vi "Start SSH Module.vi"(7 "Run as Singleton? (F)":bool, 8 "error in (no error)":errorcluster, 10 "Connection Info":T1={"host IP"="", "port"=22, "username"="lanforge", "password"="lanforge", "Connection Name"=""}) -> (0 "error out":errorcluster, 2 "Module ID":i32, 5 "SSH Broadcast Events":T2)   [LabVIEW 2017]
doc: "Creates a new instance of an SSH client with the login details specified.\nIf \"Run as Singleton\" is set to true, only one instance of the client may be created.\nRecord \"SSH Broadcast Events\" if you want to register for updates from the SSH client.\nRecord Module ID (or Connection Name) to talk to the module in future."
uses:
  Libraries/SSH/Did Init Argument--cluster.ctl
  Libraries/SSH/Status Updated Argument--cluster.ctl
  Libraries/SSH/Error Reported Argument--cluster.ctl
  Libraries/SSH/Stop Argument--cluster.ctl
  Libraries/SSH/Get Module Execution Status Argument--cluster.ctl
  Libraries/SSH/Connection Info.ctl
  Libraries/SSH/SSH.lvlib
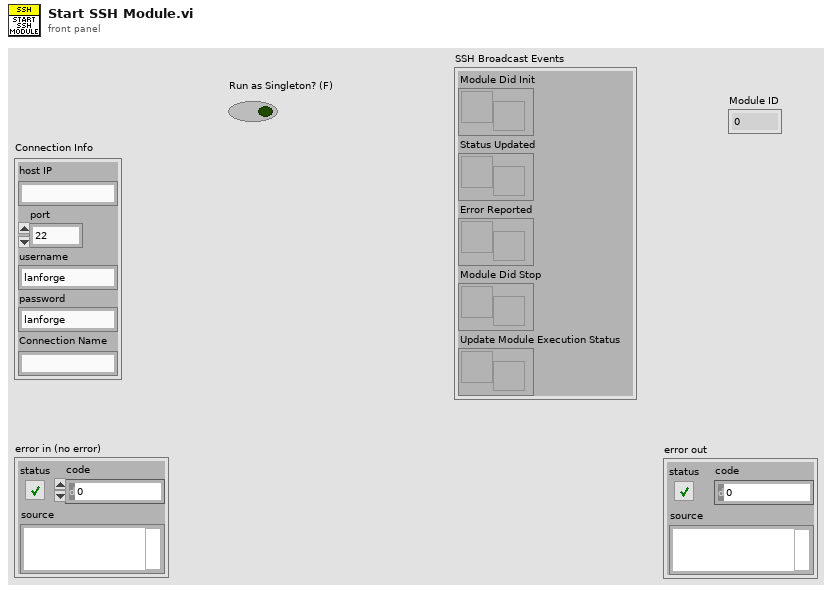
[diagram p1: front panel]
types:
  T1 = typedef "SSH.lvlib/Connection Info.ctl" = cluster{"host IP":string, "port":i32, "username":string, "password":string, "Connection Name":string}
  T2 = cluster{"Module Did Init":refnum<user-event>, "Status Updated":refnum<user-event>, "Error Reported":refnum<user-event>, "Module Did Stop":refnum<user-event>, "Update Module Execution Status":refnum<user-event>}
  T3 = typedef "SSH.lvlib/Broadcast Events--cluster.ctl" = cluster{"Module Did Init":refnum<user-event>, "Status Updated":refnum<user-event>, "Error Reported":refnum<user-event>, "Module Did Stop":refnum<user-event>, "Update Module Execution Status":refnum<user-event>}
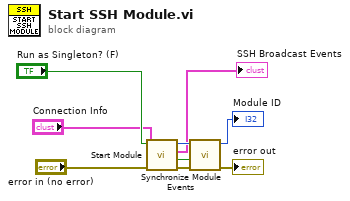
[diagram p0: block diagram]
diagram:
  n1 = call "Start Module.vi"("error in (no error)"="error in (no error)", "Connection Info"="Connection Info", "Run as Singleton? (F)"="Run as Singleton? (F)") -> ("error out"=w8:errorcluster, "Wait for Event Sync?"=w7:bool, "SSH Broadcast Events"=→"SSH Broadcast Events":T3, "Module ID"=w9:i32)  [unwired: 5 in]
  n2 = call "Synchronize Module Events.vi"("error in (no error)"=w8, "Wait for Event Sync?"=w7, "Module ID"=w9) -> ("error out"=→"error out":errorcluster, "Module ID (dup)"=→"Module ID":i32)  [unwired: 7 in]
